vi "ProgMon.TEST - Progress Monitor.vi"() -> ()   [LabVIEW 2024, in "EQMF.lvlib" / "Status Utils.lvlib"]
uses:
  Status Utils.lvlib
  PrgMon.Action.ctl
panel:
  in  "Resume":bool
  in  "Suspend":bool
  in  "stop":bool
  out "% Complete":dbl(slide) scale=0.0..1.0
  out "Expected Completion":string
  in  "Rem Secs":dbl
  in  "Est Rem Sec":bool
  in  "End":bool
  in  "Start":bool
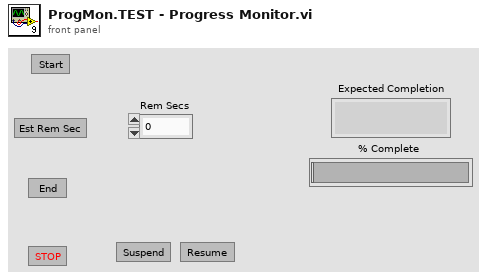
[diagram p1: front panel]
types:
  T1 = typedef "EQMF.lvlib/Status Utils.lvlib/PrgMon.Action.ctl" = enum16{"Reset", "Start", "Set Rem Secs", "Suspend", "Resume", "End"}
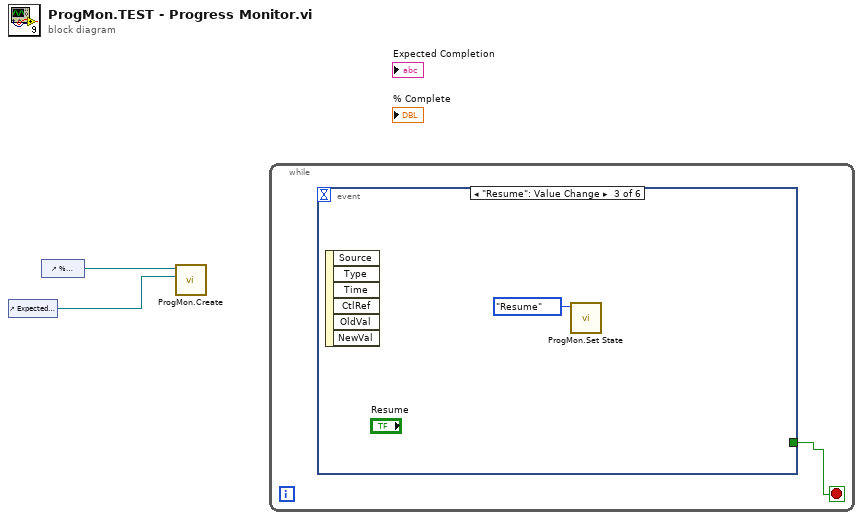
[diagram p0: block diagram]
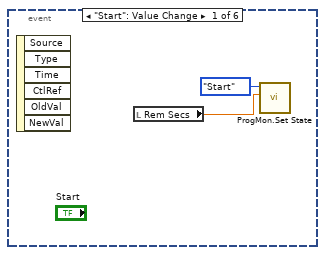
[diagram p2: hidden frame]
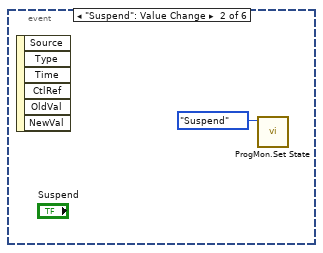
[diagram p3: hidden frame]
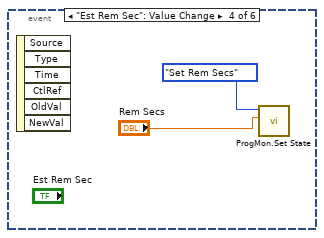
[diagram p4: hidden frame]
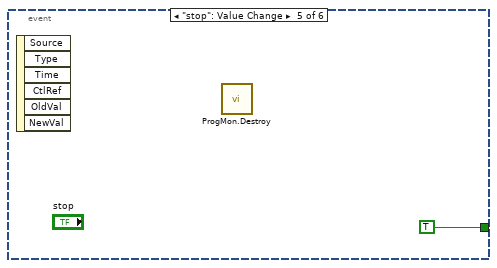
[diagram p5: hidden frame]
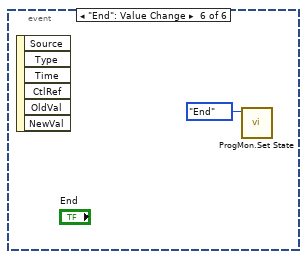
[diagram p6: hidden frame]
diagram:
  n1 = control-ref of="Expected Completion"() -> (w1:refnum<vi>)
  n2 = control-ref of="% Complete"() -> (w2:refnum<vi>)
  n3 = call "ProgMon.Create.vi"("Ref CtrlEst"=w1, "Ref CtrlComp"=w2) -> ()  [unwired: 9 in, 1 out]
  n4 = while {
    stop <- w3 stop-if-true
    n5 = event shown="[2] \"Resume\": Value Change" {
      selector: _ -> [_ _ _ _ _ _]
      dyn-events: _ -> [_ _ _ _ _ _]
      timeout: _ -> [_ _ _ _ _ _]
      tunnel: [_ _ _ _ TRUE _] -> w3
      event "Start": Value Change {
        n6 = event-data() -> ()  [unwired: 1 in, 6 out]
        n7 = local read "Rem Secs"() -> (w4:dbl)
        n8 = call "ProgMon.Set State.vi"("Remaining Secs"=w4, "Action"=PrgMon.Action."Start") -> ()  [unwired: 9 in, 1 out]
      }
      event "Suspend": Value Change {
        n9 = event-data() -> ()  [unwired: 1 in, 6 out]
        n10 = call "ProgMon.Set State.vi"("Action"=PrgMon.Action."Suspend") -> ()  [unwired: 10 in, 1 out]
      }
      event "Resume": Value Change {
        n11 = event-data() -> ()  [unwired: 1 in, 6 out]
        n12 = call "ProgMon.Set State.vi"("Action"=PrgMon.Action."Resume") -> ()  [unwired: 10 in, 1 out]
      }
      event "Est Rem Sec": Value Change {
        n13 = event-data() -> ()  [unwired: 1 in, 6 out]
        n14 = call "ProgMon.Set State.vi"("Remaining Secs"="Rem Secs", "Action"=PrgMon.Action."Set Rem Secs") -> ()  [unwired: 9 in, 1 out]
      }
      event "stop": Value Change {
        n15 = event-data() -> ()  [unwired: 1 in, 6 out]
        n16 = call "ProgMon.Destroy.vi"() -> ()  [unwired: 11 in, 1 out]
      }
      event "End": Value Change {
        n17 = event-data() -> ()  [unwired: 1 in, 6 out]
        n18 = call "ProgMon.Set State.vi"("Action"=PrgMon.Action."End") -> ()  [unwired: 10 in, 1 out]
      }
    }
  }
